vi "Moving Average.vi"() -> ()   [LabVIEW 2023]
doc: "This example shows how to perform moving average or linear filter on a univariate time series with the TSA Moving Average VI.\n\n<b>Instructions</b>\n1) Run this VI.\n2) Select the moving average method and observe the result."
uses:
  <vilib>/addons/Time Series Analysis/Utilities.llb/TSA Data.ctl
  <vilib>/addons/Time Series Analysis/Series Preprocess.llb/TSA Moving Average (Waveform).vi
  <vilib>/addons/_Advanced Signal Processing/NI_AdvSigProcTSA.lvlib
panel:
  in  "stop":bool
  in  "Method":u16(ring)=1 items=["Spencer (15 term)"=1, "Henderson (7 term)"=2, "Henderson (9 term)"=3, "Henderson (13 term)"=4, "Henderson (23 term)"=5]
  out "Period Product Sales":waveform(dbl)[](graph)
  # "Overview: Shows how to perform moving average or linear filter on a univariate time series with the TSA Moving Average VI.\nRequirements: LabVIEW Full Development System, Advanced Signal Processing Toolkit\nInstructions: \n1. Run this VI.\n2. Select the moving average method and observe the result.\n3. Click Stop to stop the VI."
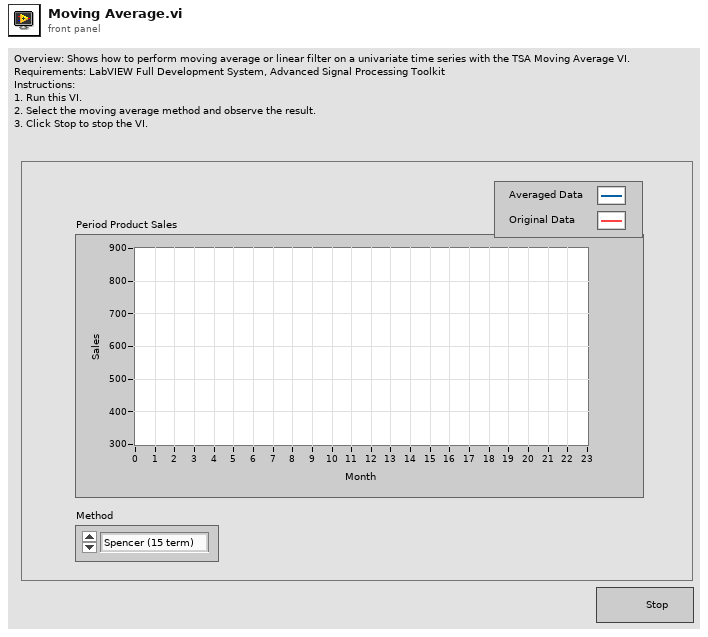
[diagram p1: front panel]
types:
  T1 = typedef "NI_AdvSigProcTSA.lvlib/TSA Data.ctl" = u16
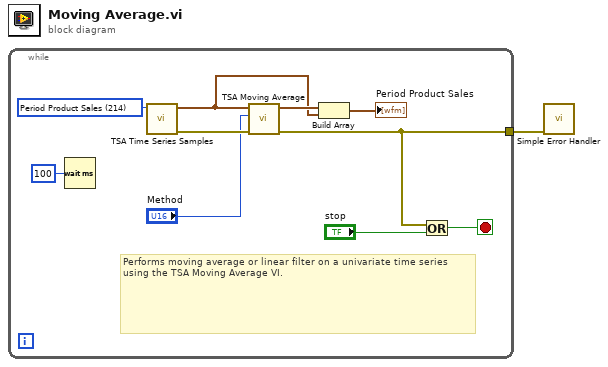
[diagram p0: block diagram]
diagram:
  n1 = while {
    tunnel: [w2] -> w1
    stop <- w4 stop-if-true
    w3 = T1 214 items=["Kobe Earthquake"=201, "EEG"=210, "Bearing Vibration (simulated)"=211, "Period Product Sales"=214, "Beam Vibration (nonlinear)"=217, "Beam Vibration (linear)"=218, "Signal With Echo"=219, "Engine Knocking"=220, "Power Line"=221, "-"=200, "Beam Deflections (multivariate)"=207, "Structure Vibration (multivariate)"=208, "Human MEG (multivariate)"=222] ("data")
    # "Performs moving average or linear filter on a univariate time series using the TSA Moving Average VI."
    n2 = Wait (ms)(milliseconds to wait=u32 100 ("millisecond multiple")) -> ()  [unwired: 1 out]
    n3 = call <vilib>:"TSA Time Series Samples.vi"("data"=w3) -> ("error out"=w10:errorcluster, "univariate time series"=w7:waveform(dbl))  [unwired: 1 in, 8 out]
    n4 = call-poly <vilib>:"TSA Moving Average.vi"("error in (no error)"=w10, "method"="Method", "Xt"=w7) -> ("error out"=w2:errorcluster, "Xt out"=w8:waveform(dbl))  [unwired: 7 out]
    n5 = Build Array(w8, w7) -> (→"Period Product Sales":waveform(dbl)[])
    n6 = Or(x=w2, y="stop") -> (x .or. y?=w4:bool)
  }
  n7 = call <vilib>:"Simple Error Handler.vi"("error in (no error)"=w1) -> ()  [unwired: 1 in, 8 out]
